vi "Voltage.vi"() -> ()   [LabVIEW 2020]
uses:
  <vilib>/Analysis/baseanly.llb/Mean (DBL).vi
  Globals.vi
  <vilib>/Analysis/NI_AALBase.lvlib
panel:
  out "Meter":dbl(knob) scale=0.0..10.0
  in  "stop (F)":bool
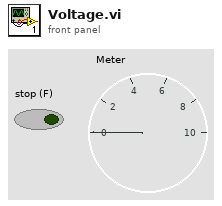
[diagram p1: front panel]
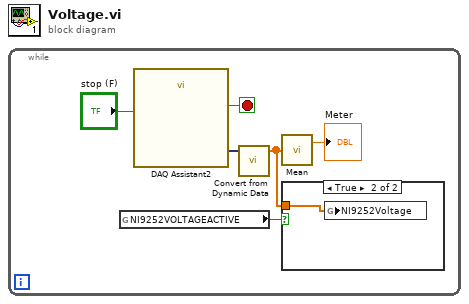
[diagram p0: block diagram]
diagram:
  n1 = while {
    stop <- w2 stop-if-true
    n2 = global read "Globals.vi" "NI9252VOLTAGEACTIVE"() -> (w4:bool)
    n3 = call "DAQ Assistant2"("stop (F)"="stop (F)") -> ("data"=w3:dynamicdata, "stopped"=w2:bool)  [unwired: 15 in, 2 out]
    n4 = call "Convert from Dynamic Data"("Dynamic Data Type"=w3) -> ("Array"=w5:dbl[])  [unwired: 3 in]
    n5 = call-poly <vilib>:"Mean.vi"("X"=w5) -> ("mean"=→"Meter":dbl)  [unwired: 1 out]
    n6 = case shown="True" w4 {
      tunnel: w5 -> [_ w7]
      frame False {
      }
      frame True {
        n7 = global write "Globals.vi" "NI9252Voltage"(w7) -> ()
      }
    }
  }
